vi "switchRelays.vi"(11 "controlRelays":u8) -> (3 "debugControlRelays":u8)   [LabVIEW 2018]
doc: "This VI will interact with the cRIO outputs, driving 24 Volts relays."
uses:
  <vilib>/rvi/eio/common/nirviEmuTemplateMethod_errors.vi
  <vilib>/eio/EIONode/EIONode.xnode
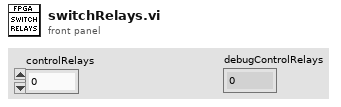
[diagram p1: front panel]
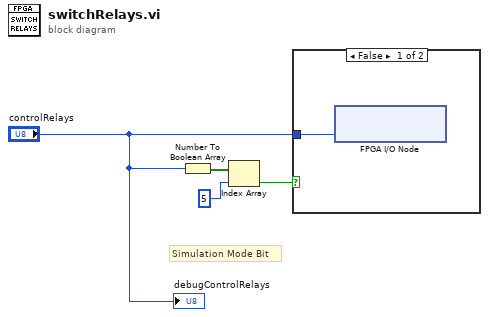
[diagram p0: block diagram]
diagram:
  # "Simulation Mode Bit"
  n1 = Number To Boolean Array(number="controlRelays") -> (Boolean array=w3:bool[])
  n2 = Index Array(array=w3, index=5) -> (element=w1:bool)
  n3 = case shown="False" w1 {
    tunnel: "controlRelays" -> [w5 _]
    frame False {
      n4 = xnode "FPGA I/O Node"("Mod4/CH7:0"=w5) -> ()  [unwired: 1 in, 1 out]
    }
    frame True {
      # "Simulation Mode On"
    }
  }
  "debugControlRelays" <- "controlRelays"
